vi "Probe.vi"() -> ()   [LabVIEW 2013]
panel:
  in  "stop":bool
  out "x > y?":bool
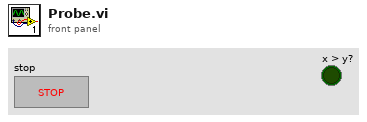
[diagram p1: front panel]
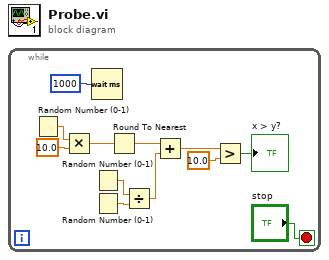
[diagram p0: block diagram]
diagram:
  n1 = while {
    stop <- "stop" stop-if-true
    n2 = Random Number (0-1)() -> (number: 0 to 1=w12:dbl)
    n3 = Multiply(x=w12, y=10.0) -> (x*y=w10:dbl)
    n4 = Wait (ms)(milliseconds to wait=u32 1000) -> ()  [unwired: 1 out]
    n5 = Random Number (0-1)() -> (number: 0 to 1=w9:dbl)
    n6 = Random Number (0-1)() -> (number: 0 to 1=w8:dbl)
    n7 = Round To Nearest(number=w10) -> (nearest integer value=w7:dbl)
    n8 = Divide(x=w9, y=w8) -> (x/y=w6:dbl)
    n9 = Add(x=w7, y=w6) -> (x+y=w5:dbl)
    n10 = Greater?(x=w5, y=10.0) -> (0:→"x > y?":bool)
  }
